vi "test-Ellip-Region-Constraint-Test1.vi"(8 "error in (no error)":errorcluster) -> (0 "error out":errorcluster, 3 "All tests passed":bool)   [LabVIEW 2019]
uses:
  <vilib>/Rock Robotics/WPI/ThirdParty/JAS_Junk/TrajLib/TRAJECTORY.ctl
  <vilib>/Rock Robotics/WPI/ThirdParty/JAS_Junk/TrajLib/TRAJ_STATE.ctl
  <vilib>/Rock Robotics/WPI/ThirdParty/JAS_Junk/TrajLib/POSE2D.ctl
  <vilib>/Rock Robotics/WPI/ThirdParty/JAS_Junk/TrajLib/TRANSLATION2D.ctl
  <vilib>/Rock Robotics/WPI/ThirdParty/JAS_Junk/TrajLib/ROTATION2D.ctl
  <vilib>/Rock Robotics/WPI/ThirdParty/JAS_Junk/TrajLib/TRAJ_CONFIG.ctl
  <vilib>/Rock Robotics/WPI/ThirdParty/JAS_Junk/TrajLib/TypeDef/TRAJ_CONSTRAINT_ELLIP_REGION.ctl
  <vilib>/Rock Robotics/WPI/ThirdParty/JAS_Junk/TrajLib/Enum/TRAJ_CONSTRAINT_TYPES_ENUM.ctl
  <vilib>/Rock Robotics/WPI/ThirdParty/JAS_Junk/TrajLib/Conv_Deg_Radians.vi
  <vilib>/Rock Robotics/WPI/ThirdParty/JAS_Junk/TrajLib/Rotation2d_CreateAngle.vi
  <vilib>/Rock Robotics/WPI/ThirdParty/JAS_Junk/TrajLib/VI/TrajConstraint_GetType.vi
  <vilib>/Rock Robotics/WPI/ThirdParty/JAS_Junk/TrajLib/Translation2d_RotateBy.vi
  <vilib>/Utility/Data Type/Get Type Information.vi
  <vilib>/Rock Robotics/WPI/ThirdParty/JAS_Junk/TrajLib/Trajectory_Library.lvlib
panel:
  out "XY Graph   --- FEET":cluster{dbl[], dbl[]}(graph)
  out "ELLIP_REGION_CONSTRAINT":T1={"Center"={"X"=0.0, "Y"=0.0}, "Radii"={"X"=0.0, "Y"=0.0}, "Constraint"=variant, "Constraint Type"=enum."DIFF DRIVE KINEMATICS", "IM UNIQUE"=FALSE} {"Radii"."Y" format="%14.3f"; "Radii"."X" format="%14.3f"; "Center"."Y" format="%14.3f"; "Center"."X" format="%14.3f"}
  out "Was in region":bool
  out "Didnt Exceed Inside":bool
  out "Exceeded outside":bool
  out "outTRAJECTORY_CONFIG":T4 {"End Velocity" format="%20.4f"; "StartVelocity" format="%20.4f"; "Max Acceleration" format="%20.4f"; "MaxVelocity" format="%20.4f"}
  out "PoseInRegion":bool
  out "error out 2":errorcluster
  out "TRAJECTORY":T5 {"States"."POSE"."ROTATION"."SIN" format="%13.4f"; "States"."POSE"."ROTATION"."COS" format="%13.4f"; "States"."POSE"."ROTATION"."VALUE" format="%13.4f"; "States"."POSE"."TRANSLATION"."Y" format="%14.3f"; "States"."POSE"."TRANSLATION"."X" format="%14.3f"; "TotalTImeSecs" format="%20.3f"}
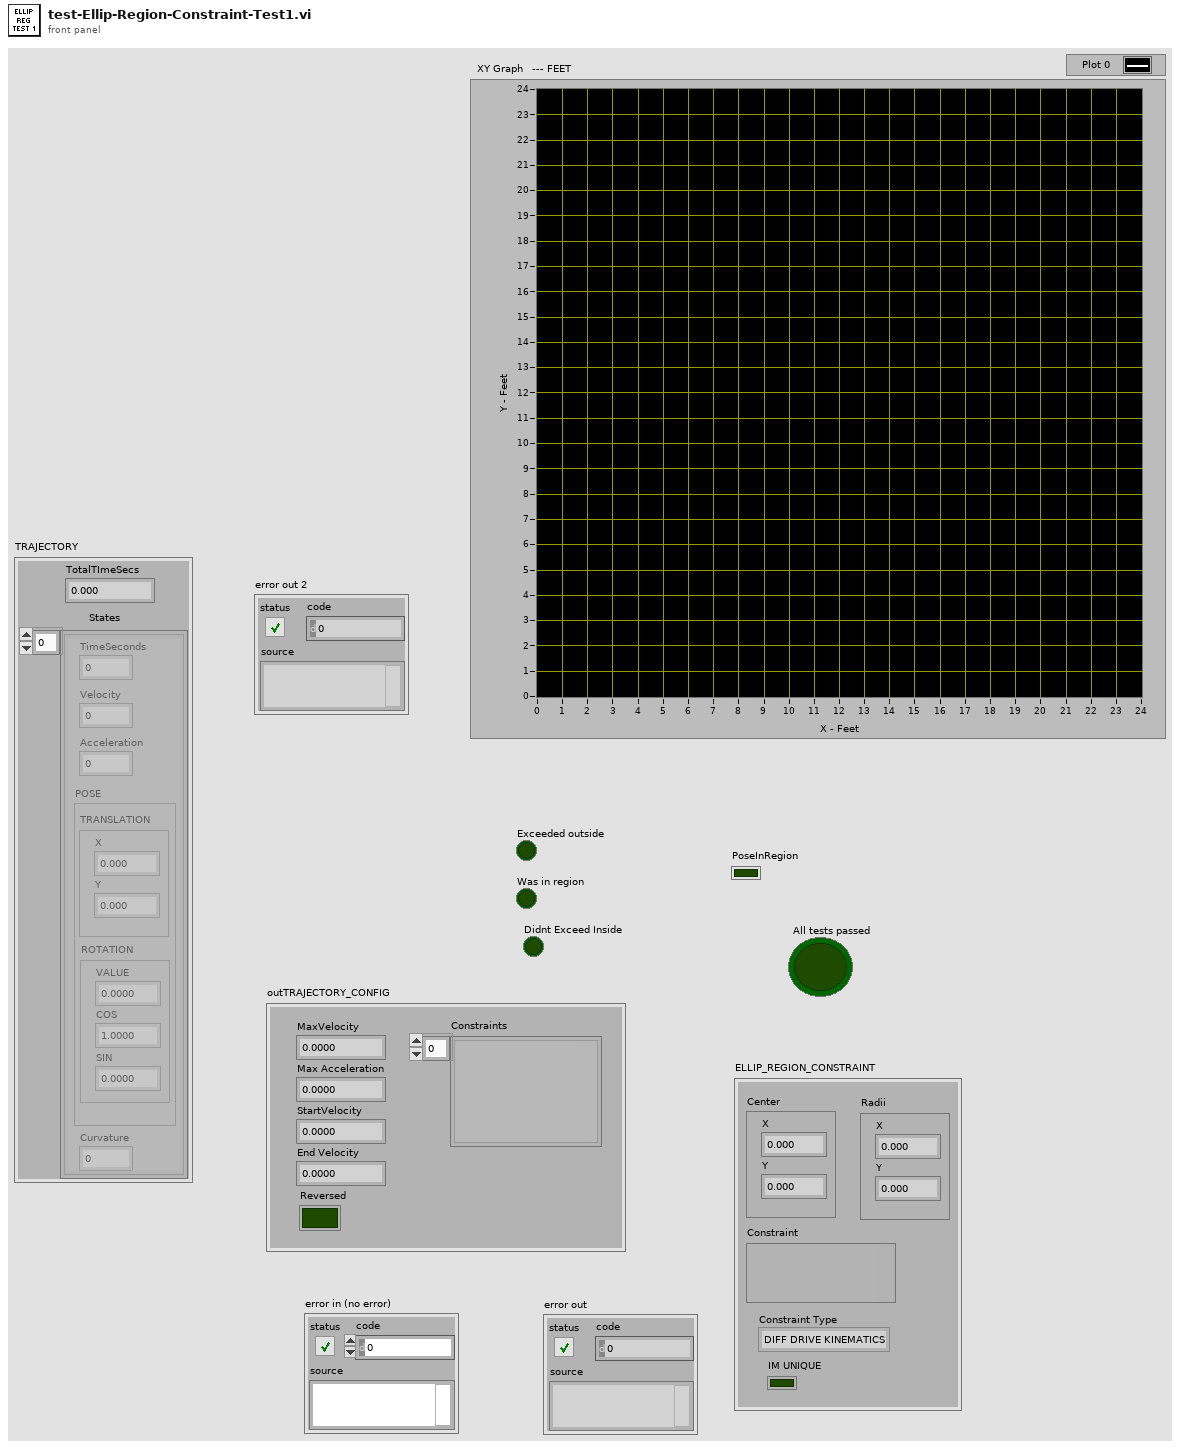
[diagram p1: front panel]
types:
  T1 = typedef "Trajectory_Library.lvlib/TRAJ_CONSTRAINT_ELLIP_REGION.ctl" = cluster{"Center":T2, "Radii":T2, "Constraint":variant, "Constraint Type":T3, "IM UNIQUE":bool}
  T2 = typedef "Trajectory_Library.lvlib/TRANSLATION2D.ctl" = cluster{"X":dbl, "Y":dbl}
  T3 = typedef "Trajectory_Library.lvlib/TRAJ_CONSTRAINT_TYPES_ENUM.ctl" = enum16{"UNDEFINED", "DIFF DRIVE KINEMATICS", "DIFF DRIVE VOLTAGE", "CENTRIPITAL ACCEL", "MECA DRIVE KINEMATICS", "SWERVE DRIVE KINEMATICS", "MAXIMUM VELOCITY", "ELLIPTICAL REGION", "RECTANGULAR REGION"}
  T4 = typedef "Trajectory_Library.lvlib/TRAJ_CONFIG.ctl" = cluster{"MaxVelocity":dbl, "Max Acceleration":dbl, "StartVelocity":dbl, "End Velocity":dbl, "Reversed":bool, "Constraints":variant[]}
  T5 = typedef "Trajectory_Library.lvlib/TRAJECTORY.ctl" = cluster{"TotalTImeSecs":dbl, "States":T6[]}
  T6 = typedef "Trajectory_Library.lvlib/TRAJ_STATE.ctl" = cluster{"TimeSeconds":dbl, "Velocity":dbl, "Acceleration":dbl, "POSE":T7, "Curvature":dbl}
  T7 = typedef "Trajectory_Library.lvlib/POSE2D.ctl" = cluster{"TRANSLATION":T2, "ROTATION":T8}
  T8 = typedef "Trajectory_Library.lvlib/ROTATION2D.ctl" = cluster{"VALUE":dbl, "COS":dbl, "SIN":dbl}
  T9 = typedef "Trajectory_Library.lvlib/TRAJ_CONSTRAINT_MAX_VELOCITY.ctl" = cluster{"Max Velocity":dbl, "IM UNIQUE":bool}
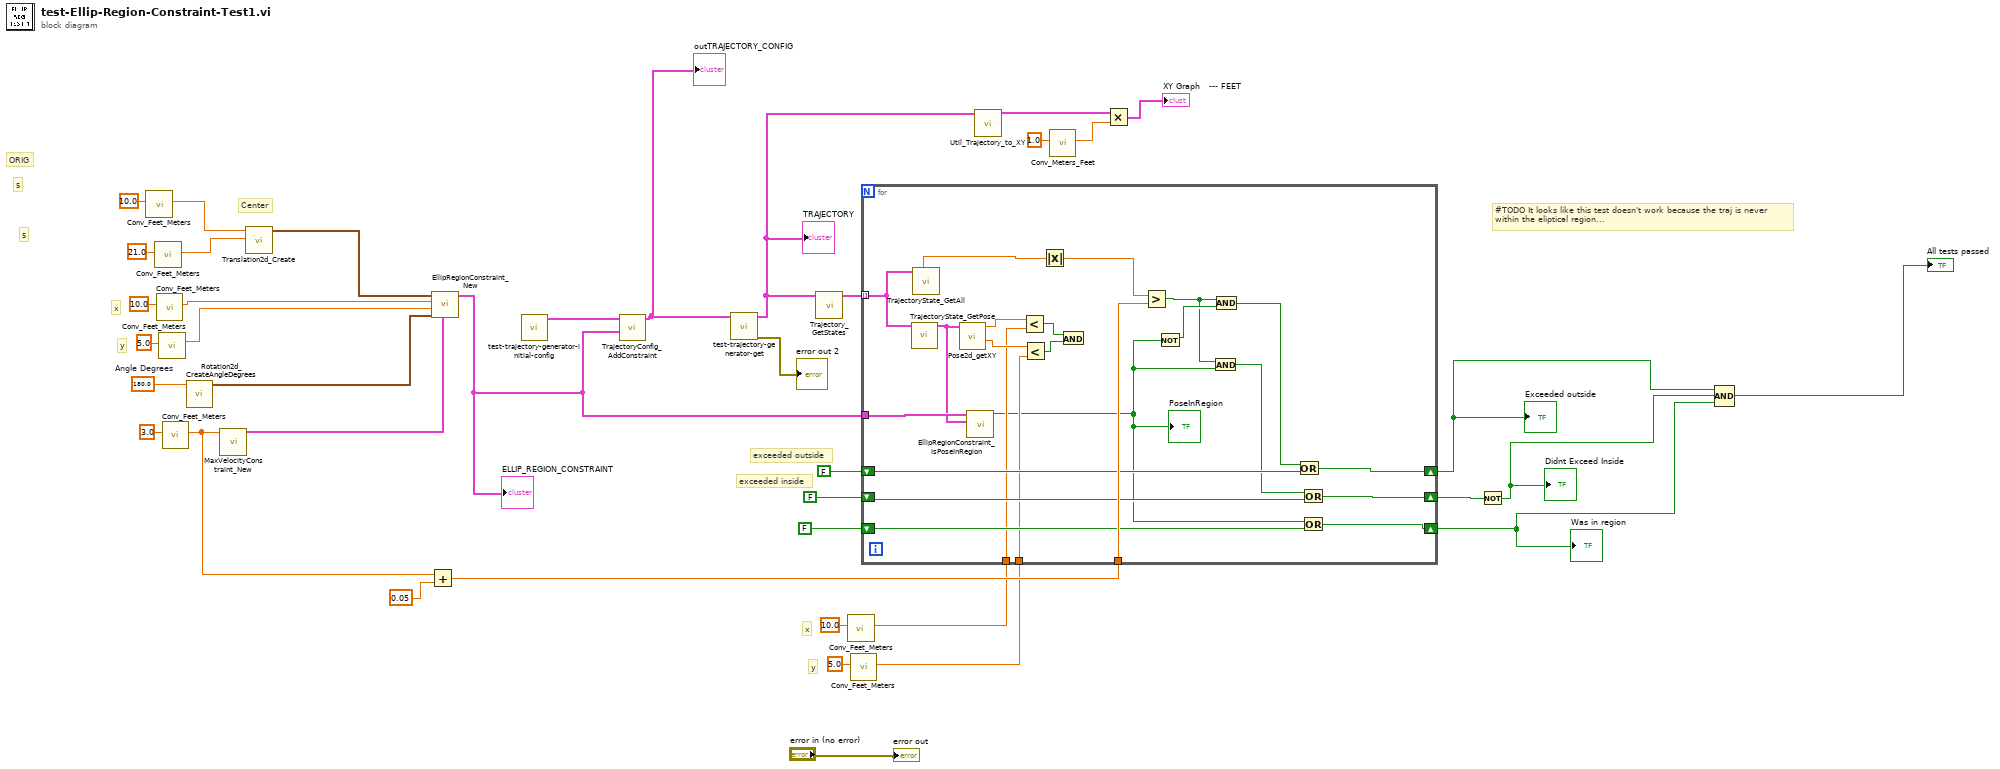
[diagram p0: block diagram]
diagram:
  w14 = 180.0  # Angle Degrees
  # "5"
  # "5"
  # "ORIG"
  # "#TODO It looks like this test doesn't work because the traj is never\nwithin the eliptical region..."
  # "y"
  # "x"
  # "y"
  # "x"
  # "Center"
  # "exceeded inside"
  # "exceeded outside"
  n1 = call <vilib>:"Conv_Feet_Meters.vi"("Feet"=10.0) -> ("Meters"=w19:dbl)  [unwired: 10 in]
  n2 = call <vilib>:"Conv_Feet_Meters.vi"("Feet"=21.0) -> ("Meters"=w18:dbl)  [unwired: 10 in]
  n3 = call <vilib>:"Conv_Feet_Meters.vi"("Feet"=10.0) -> ("Meters"=w16:dbl)  [unwired: 10 in]
  n4 = call <vilib>:"Conv_Feet_Meters.vi"("Feet"=5.0) -> ("Meters"=w15:dbl)  [unwired: 10 in]
  n5 = call <vilib>:"Conv_Feet_Meters.vi"("Feet"=3.0) -> ("Meters"=w12:dbl)  [unwired: 10 in]
  n6 = call <vilib>:"Rotation2d_CreateAngleDegrees.vi"("Angle_Degrees"=w14) -> ("ROTATION"=w13:T8)  [unwired: 10 in]
  n7 = call <vilib>:"MaxVelocityConstraint_New.vi"("Maximum Velocity"=w12) -> ("MAX_VELOCITY_CONSTRAINT"=w17:T9)  [unwired: 10 in]
  n8 = call <vilib>:"Translation2d_Create.vi"("Y"=w18, "X"=w19) -> ("TRANSLATION"=w24:T2)  [unwired: 9 in]
  n9 = Add(x=w12, y=0.05) -> (x+y=w33:dbl)
  n10 = call <vilib>:"EllipRegionConstraint_New.vi"("Constraint Data Cluster"=w17, "Rotation"=w13, "Y Width"=w15, "X Width"=w16, "Center"=w24) -> ("ELLIP_REGION_CONSTRAINT"=w11:T1)  [unwired: 6 in]
  "ELLIP_REGION_CONSTRAINT" <- w11
  n11 = call "test-trajectory-generator-initial-config.vi"() -> ("traj_config"=w38:T4)  [unwired: 11 in]
  n12 = call <vilib>:"TrajectoryConfig_AddConstraint.vi"("Constraint"=w11, "inTRAJECTORY_CONFIG"=w38) -> ("outTRAJECTORY_CONFIG"=w6:T4)  [unwired: 9 in]
  "outTRAJECTORY_CONFIG" <- w6
  n13 = call "test-trajectory-generator-get.vi"("traj_config"=w6) -> ("error out"=→"error out 2":errorcluster, "TRAJECTORY"=w5:T5)  [unwired: 8 in, 1 out]
  "TRAJECTORY" <- w5
  n14 = call <vilib>:"Trajectory_GetStates.vi"("TRAJECTORY"=w5) -> ("States"=w36:T6[])  [unwired: 10 in]
  n15 = call <vilib>:"Conv_Feet_Meters.vi"("Feet"=10.0) -> ("Meters"=w8:dbl)  [unwired: 10 in]
  n16 = call <vilib>:"Conv_Feet_Meters.vi"("Feet"=5.0) -> ("Meters"=w7:dbl)  [unwired: 10 in]
  n17 = for {
    tunnel: w36 -> [w61] mode=indexing
    tunnel: w11 -> [w62]
    shift-right: [w60] -> w30
    shift-left: FALSE -> [w54]
    tunnel: w33 -> [w57]
    shift-right: [w50] -> w29
    shift-left: FALSE -> [w51]
    shift-right: [w48] -> w27
    shift-left: FALSE -> [w49]
    tunnel: w8 -> [w44]
    tunnel: w7 -> [w43]
    n18 = call <vilib>:"TrajectoryState_GetPose.vi"("TRAJ_STATE"=w61) -> ("TrajStatePose"=w47:T7)  [unwired: 10 in]
    n19 = call <vilib>:"TrajectoryState_GetAll.vi"("TRAJ_STATE"=w61) -> ("Velocity"=w59:dbl)  [unwired: 4 in, 6 out]
    n20 = call <vilib>:"Pose2d_getXY.vi"("in POSE"=w47) -> ("Y"=w45:dbl, "X"=w46:dbl)  [unwired: 9 in]
    n21 = call <vilib>:"EllipRegionConstraint_IsPoseInRegion.vi"("statePose"=w47, "ELLIP_REGION_CONSTRAINT"=w62) -> ("PoseInRegion"=w40:bool)  [unwired: 9 in]
    "PoseInRegion" <- w40
    n22 = Less?(x=w46, y=w44) -> (x < y?=w41:bool)
    n23 = Less?(x=w45, y=w43) -> (x < y?=w42:bool)
    n24 = Absolute Value(x=w59) -> (abs(x)=w58:dbl)
    n25 = And(x=w41, y=w42) -> ()  [unwired: 1 out]
    n26 = Greater?(x=w58, y=w57) -> (0:w53:bool)
    n27 = Not(x=w40) -> (.not. x?=w56:bool)
    n28 = And(x=w53, y=w40) -> (x .and. y?=w52:bool)
    n29 = And(x=w53, y=w56) -> (x .and. y?=w55:bool)
    n30 = Or(x=w55, y=w54) -> (x .or. y?=w60:bool)
    n31 = Or(x=w52, y=w51) -> (x .or. y?=w50:bool)
    n32 = Or(x=w40, y=w49) -> (x .or. y?=w48:bool)
  }
  "Exceeded outside" <- w30
  "Was in region" <- w27
  n33 = call <vilib>:"Util_Trajectory_to_XY.vi"("TRAJECTORY"=w5) -> ("outArrayXY"=w4:cluster{dbl[], dbl[]})  [unwired: 10 in]
  n34 = call <vilib>:"Conv_Meters_Feet.vi"("Meters"=1.0) -> ("Feet"=w2:dbl)  [unwired: 10 in]
  n35 = Multiply(x=w4, y=w2) -> (x*y=→"XY Graph   --- FEET":cluster{dbl[], dbl[]})
  n36 = Not(x=w29) -> (.not. x?=w28:bool)
  "Didnt Exceed Inside" <- w28
  n37 = Compound Arithmetic op=AND(w30, w28, w27) -> (→"All tests passed":bool)
  "error out" <- "error in (no error)"
